vi "ClsGetNextSampleSingleChannelDevice.vi"(8 "error in (no error)":errorcluster, 11 "Connection In":u32) -> (0 "error out":errorcluster, 1 "Number Of Signals out":i32, 2 "Data":dbl[](array[numeric]), 3 "Connection Out":u32, 5 "Have Data?":bool)   [LabVIEW 2015]
doc: "Get Next Sample:\n\nThis function is used for single channel devices. This function is used to get the next valid sample from device. If client does not use any data reading, buffer flushing or command sennding subVIs frequent enough, client will be out of sync of the data buffer. In this case, this function can fail. Client can go back to sync with data buffer by jumping to the last valid position (start position of the last unfinished telegram) in the buffer by calling function “FlushInputBuffer”. Note that this function is none-block which means it will return immediately no matter if there is any data available.\n\nConnection In[Input]: the connection handle which is initially created by Open Connection subVI.\n\nHave data?[Output]: since this subVI is none-block which will return immediately with an empty data array if there is no data available, this boolean output is used for indicating whether there is any data in the output at all.\n\nData[Output]: The one dimensional array for data. Note that you can use Get Signal IDs subVI to see the ordering of signal IDs corresponding to this data array. If there is no data, an empty array will be returned.\n\nConnection Out[Output]: the connection handle output which could be used for next subVI refering to the same connection."
uses:
  dependent dlls/CHRocodileDLL.dll
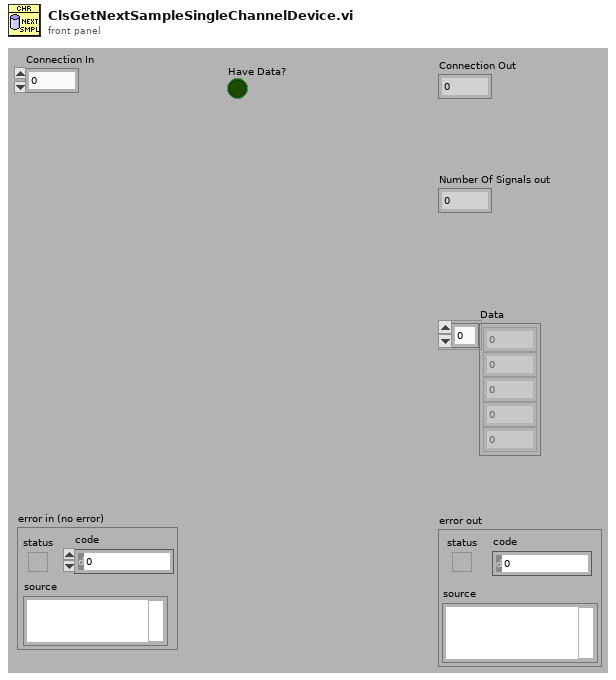
[diagram p1: front panel]
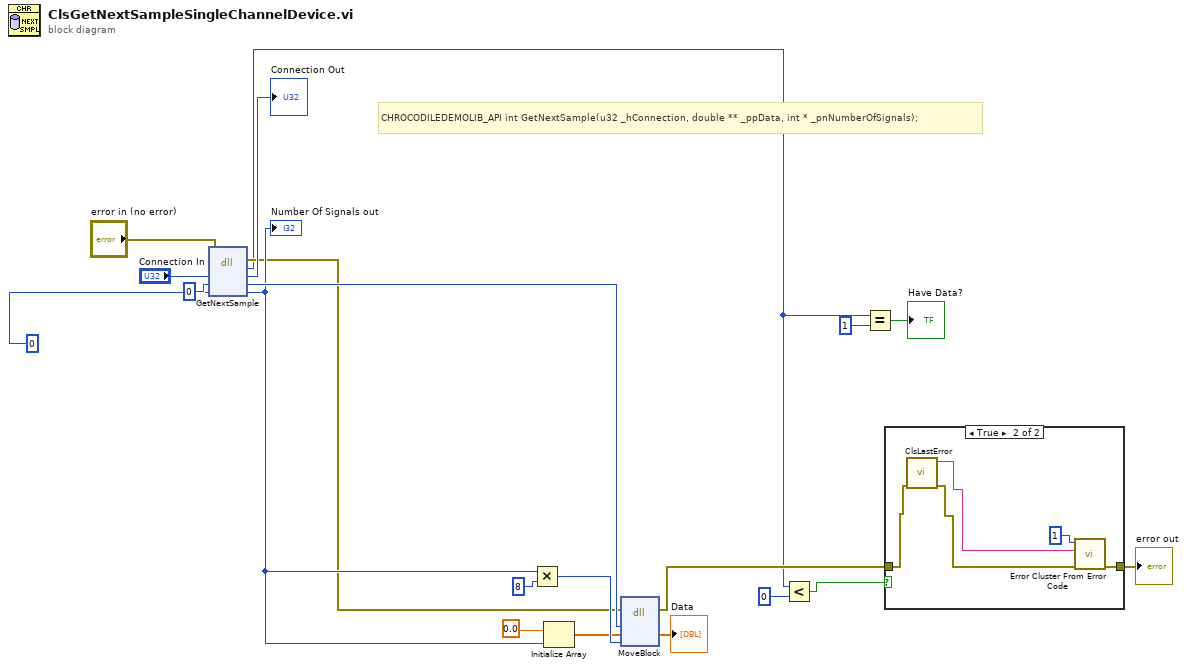
[diagram p0: block diagram]
diagram:
  # "CHROCODILEDEMOLIB_API int GetNextSample(u32 _hConnection, double ** _ppData, int * _pnNumberOfSignals);"
  n1 = dll-call lib="C:/Users/privat/Documents/ADP-SLA/Drop Impact Teststand/dependent dlls/CHRocodileDLL.dll" fn="GetNextSample"(error in="error in (no error)", "_hConnection"="Connection In", "_ppData"=i64 0, "_pnNumberOfSignals"=0) -> (error out=w9:errorcluster, "return type"=w3:i32, "_hConnection"=→"Connection Out":u32, "_ppData"=w18:i64, "_pnNumberOfSignals"=w13:i32)  [unwired: 2 in, 1 out]
  "Number Of Signals out" <- w13
  n2 = Multiply(x=w13, y=8) -> (x*y=w15:i32)
  n3 = Initialize Array(0.0, w13) -> (w12:dbl[])
  n4 = dll-call lib="LabVIEW" fn="MoveBlock"(error in=w9, "Address(pointer)"=w18, "Destination"=w12, "Size"=w15) -> (error out=w4:errorcluster, "Destination"=→"Data":dbl[])  [unwired: 5 in, 1 out]
  n5 = Less?(x=w3, y=0) -> (x < y?=w5:bool)
  n6 = Equal?(x=w3, y=1) -> (x = y?=→"Have Data?":bool)
  n7 = case shown="True" w5 {
    tunnel: [w21 w25] -> w7
    tunnel: w4 -> [w21 w24]
    frame False {
    }
    frame True {
      n8 = call "ClsLastError.vi"("error in (no error)"=w24) -> ("error out"=w23:errorcluster, "Error Message"=w22:string)  [unwired: 9 in]
      n9 = call <vilib>:"Error Cluster From Error Code.vi"("error in (no error)"=w23, "error message (\"\")"=w22, "error code (0)"=1) -> ("error out"=w25:errorcluster)  [unwired: 6 in]
    }
  }
  "error out" <- w7
